vi "Measure.vi"(10 "t (seconds)":dbl, 11 "Sine in":refnum<class "Sine.lvclass">) -> (2 "y":dbl, 3 "Sine out":refnum<class "Sine.lvclass">)   [LabVIEW 2020, in "Sine.lvclass"]
uses:
  Sine.lvclass
  Sine.lvclass/Sine.ctl
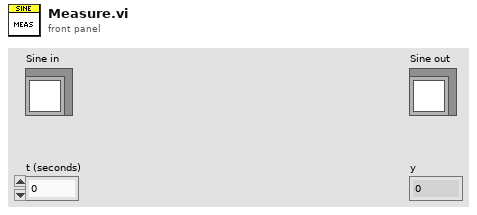
[diagram p1: front panel]
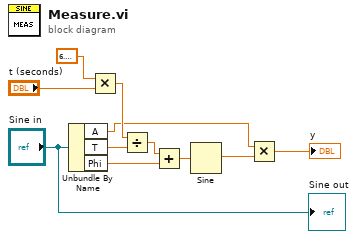
[diagram p0: block diagram]
diagram:
  n1 = Unbundle By Name("Sine in") -> ("A"=w2:dbl, "T"=w7:dbl, "Phi"=w5:dbl)
  n2 = Multiply(x=6.283185307179586, y="t (seconds)") -> (x*y=w8:dbl)
  n3 = Divide(x=w8, y=w7) -> (x/y=w6:dbl)
  n4 = Add(x=w6, y=w5) -> (x+y=w4:dbl)
  n5 = Sine(x=w4) -> (sin(x)=w3:dbl)
  n6 = Multiply(x=w2, y=w3) -> (x*y=→"y":dbl)
  "Sine out" <- "Sine in"
